vi "Launch Asynchronous Logging Loop.vi"(8 "error in (no error)":errorcluster, 11 "Log Data FIFO":refnum<k33>) -> (0 "error out":errorcluster)   [LabVIEW 2019, in "Inline Telemetry Prototype Engine.lvlib"]
uses:
  Inline Telemetry Prototype Engine.lvlib
  Asynchronous Logging Loop.vi
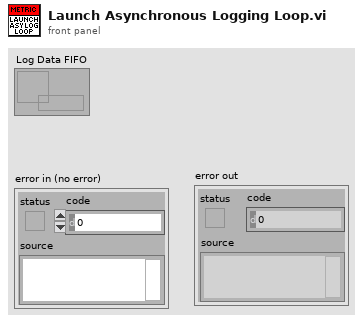
[diagram p1: front panel]
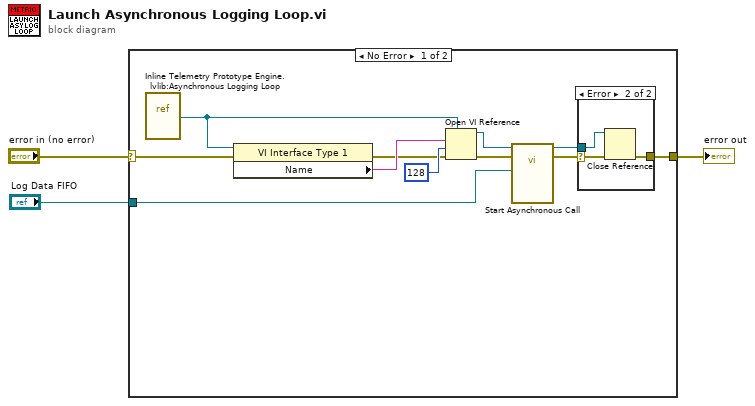
[diagram p0: block diagram]
diagram:
  n1 = case shown="No Error" "error in (no error)" {
    selector: "error in (no error)" -> [w7 w19]
    tunnel: [w13 w19] -> w3
    tunnel: "Log Data FIFO" -> [w4 _]
    frame No Error {
      n2 = vi-ref "Inline Telemetry Prototype Engine.lvlib:Asynchronous Logging Loop.vi"() -> (w5:refnum<vi>)
      n3 = property class="VI Interface Type 1"(reference=w5, error in=w7) -> (error out=w6:errorcluster, "Name"=w14:string)  [unwired: 1 out]
      n4 = Open VI Reference(type specifier VI Refnum (for type only)=w5, vi path=w14, options=128, error in (no error)=w6) -> (vi reference=w11:refnum<vi>, error out=w12:errorcluster)  [unwired: 2 out]
      n5 = call-by-ref "Start Asynchronous Call"(reference=w11, error in=w12, "Log Data FIFO"=w4) -> (reference out=w9:refnum<vi>, error out=w10:errorcluster)  [unwired: 10 in, 1 out]
      n6 = case shown="Error" w10 {
        selector: w10 -> [w15 w18]
        tunnel: w9 -> [_ w17]
        tunnel: [w15 w16] -> w13
        frame No Error {
        }
        frame Error {
          n7 = Close Reference(reference=w17, error in (no error)=w18) -> (error out=w16:errorcluster)
        }
      }
    }
    frame Error {
    }
  }
  "error out" <- w3
